vi "Main.vi"() -> ()   [LabVIEW 2019]
uses:
  Circle/Circle.lvclass
  C:/Users/RIG1/Google Drive/Projects/AMFAX/Shape/Shape.lvclass
  Square/Square.lvclass
  Shape.lvclass
panel:
  out "2D Picture":picture
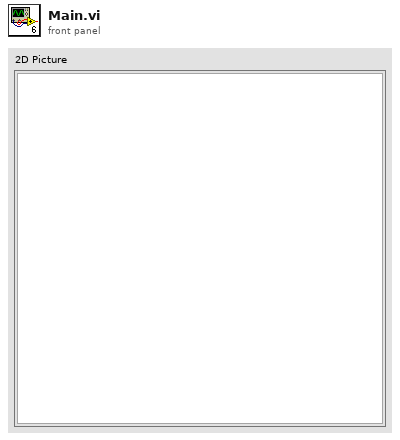
[diagram p1: front panel]
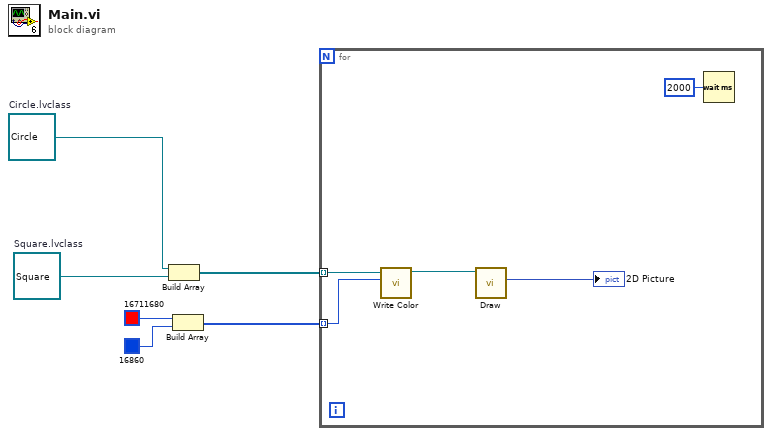
[diagram p0: block diagram]
diagram:
  w2 = refnum<class "Square.lvclass"> refnum  # Square.lvclass
  w3 = refnum<class "Circle.lvclass"> refnum  # Circle.lvclass
  n1 = Build Array(w3, w2) -> (w1:refnum<class "Shape.lvclass">[])
  n2 = Build Array(u32 16711680 ("Color Box"), u32 16860 ("Color Box")) -> (w4:u32[])
  n3 = for {
    tunnel: w4 -> [w7] mode=indexing
    tunnel: w1 -> [w10] mode=indexing
    n4 = call-dynamic "Write Color.vi"("Color"=w7, "Shape in"=w10) -> ("Shape out"=w9:refnum<class "Shape.lvclass">)  [unwired: 8 in, 1 out]
    n5 = call-dynamic "Draw.vi"("Shape in"=w9) -> ("Shape"=→"2D Picture":picture)  [unwired: 8 in, 2 out]
    n6 = Wait (ms)(milliseconds to wait=u32 2000) -> ()  [unwired: 1 out]
  }
